vi "Direct DAC Control.vi"() -> ()   [LabVIEW 2012]
uses:
  Type/_GUI Method.ctl
  Type/_Lens Property.ctl
  Type/_Mass Range Property.ctl
  Type/_Mass Range Parameters.ctl
  Type/_RT Res Type.ctl
  Type/_Run Mode.ctl
  Type/_RT Command.ctl
  Configuration/_Global Configuration.vi
panel:
  in  "Q2DC EN":bool
  in  "Count1":dbl=400.0 caption="Lens Value" format="%#.3f"
  in  "Count2":dbl=400.0 caption="High Value" format="%#.3f"
  in  "Time1":dbl=1.0 caption="Low Dwell (ms)" format="%#.3f"
  in  "Time2":dbl=1.0 caption="High Dwell (ms)" format="%#.3f"
  in  "Scans":i32=1
  in  "Step Size":dbl=-1.0 format="%#.3f"
  in  "Unit":bool
  in  "Q1DC EN":bool
  in  "Q1 POL":bool
  in  "Q2 POL":bool
  out "DAC Value":i32=98187
  in  "Lens Table":i32(listbox)
  in  "NewMethod":bool
  in  "Method":T1={"Lenses"=[{"Scan Type"=0, "Scans"=1, "Time 1"=1.0, "Time 2"=1.0, "Value 1"=400.0, "Value 2"=400.0, "Step Size"=-1.0}, {"Scan Type"=0, "Scans"=1, "Time 1"=1.0, "Time 2"=1.0, "Value 1"=150.0, "Value 2"=150.0, "Step Size"=1.0}, {"Scan Type"=0, "Scans"=1, "Time 1"=1.0, "Time 2"=1.0, "Value 1"=32000.0, "Value 2"=32000.0, "Step Size"=1.0}, {"Scan Type"=0, "Scans"=1, "Time 1"=1.0, "Time 2"=1.0, "Value 1"=400.0, "Value 2"=400.0, "Step Size"=1.0}, {"Scan Type"=0, "Scans"=1, "Time 1"=1.0, "Time 2"=1.0, "Value 1"=150.0, "Value 2"=150.0, "Step Size"=1.0}, {"Scan Type"=0, "Scans"=1, "Time 1"=1.0, "Time 2"=1.0, "Value 1"=64000.0, "Value 2"=64000.0, "Step Size"=1.0}, {"Scan Type"=0, "Scans"=1, "Time 1"=1.0, "Time 2"=1.0, "Value 1"=420.0, "Value 2"=420.0, "Step Size"=1.0}, {"Scan Type"=0, "Scans"=1, "Time 1"=1.0, "Time 2"=1.0, "Value 1"=30.0, "Value 2"=30.0, "Step Size"=1.0}, {"Scan Type"=0, "Scans"=1, "Time 1"=1.0, "Time 2"=1.0, "Value 1"=15.0, "Value 2"=15.0, "Step Size"=1.0}, {"Scan Type"=0, "Scans"=1, "Time 1"=1.0, "Time 2"=1.0, "Value 1"=0.0, "Value 2"=0.0, "Step Size"=1.0}, {"Scan Type"=0, "Scans"=1, "Time 1"=1.0, "Time 2"=1.0, "Value 1"=0.0, "Value 2"=0.0, "Step Size"=1.0}, {"Scan Type"=0, "Scans"=1, "Time 1"=1.0, "Time 2"=1.0, "Value 1"=0.0, "Value 2"=0.0, "Step Size"=1.0}, {"Scan Type"=0, "Scans"=1, "Time 1"=1.0, "Time 2"=1.0, "Value 1"=0.0, "Value 2"=0.0, "Step Size"=1.0}, {"Scan Type"=0, "Scans"=1, "Time 1"=1.0, "Time 2"=1.0, "Value 1"=0.0, "Value 2"=0.0, "Step Size"=1.0}, {"Scan Type"=0, "Scans"=1, "Time 1"=1.0, "Time 2"=1.0, "Value 1"=-0.5, "Value 2"=-0.5, "Step Size"=1.0}, {"Scan Type"=0, "Scans"=1, "Time 1"=1.0, "Time 2"=1.0, "Value 1"=-2.0, "Value 2"=-2.0, "Step Size"=1.0}, {"Scan Type"=0, "Scans"=1, "Time 1"=1.0, "Time 2"=1.0, "Value 1"=-1.2, "Value 2"=-1.2, "Step Size"=1.0}, {"Scan Type"=0, "Scans"=1, "Time 1"=1.0, "Time 2"=1.0, "Value 1"=0.0, "Value 2"=0.0, "Step Size"=1.0}, {"Scan Type"=0, "Scans"=1, "Time 1"=1.0, "Time 2"=1.0, "Value 1"=-240.0, "Value 2"=-240.0, "Step Size"=1.0}, {"Scan Type"=0, "Scans"=1, "Time 1"=1.0, "Time 2"=1.0, "Value 1"=-50.0, "Value 2"=-50.0, "Step Size"=1.0}, {"Scan Type"=0, "Scans"=1, "Time 1"=1.0, "Time 2"=1.0, "Value 1"=-52.0, "Value 2"=-52.0, "Step Size"=1.0}, {"Scan Type"=0, "Scans"=1, "Time 1"=1.0, "Time 2"=1.0, "Value 1"=-100.0, "Value 2"=-100.0, "Step Size"=1.0}, {"Scan Type"=0, "Scans"=1, "Time 1"=1.0, "Time 2"=1.0, "Value 1"=-54.0, "Value 2"=-54.0, "Step Size"=1.0}, {"Scan Type"=0, "Scans"=1, "Time 1"=1.0, "Time 2"=1.0, "Value 1"=-400.0, "Value 2"=-400.0, "Step Size"=1.0}, {"Scan Type"=0, "Scans"=1, "Time 1"=1.0, "Time 2"=1.0, "Value 1"=30.0, "Value 2"=30.0, "Step Size"=1.0}, {"Scan Type"=0, "Scans"=1, "Time 1"=1.0, "Time 2"=1.0, "Value 1"=2000.0, "Value 2"=2000.0, "Step Size"=1.0}, {"Scan Type"=0, "Scans"=1, "Time 1"=1.0, "Time 2"=1.0, "Value 1"=-6000.0, "Value 2"=-6000.0, "Step Size"=1.0}, {"Scan Type"=0, "Scans"=1, "Time 1"=1.0, "Time 2"=1.0, "Value 1"=0.0, "Value 2"=0.0, "Step Size"=1.0}, {"Scan Type"=0, "Scans"=1, "Time 1"=1.0, "Time 2"=1.0, "Value 1"=0.0, "Value 2"=0.0, "Step Size"=1.0}, {"Scan Type"=0, "Scans"=1, "Time 1"=1.0, "Time 2"=1.0, "Value 1"=250.0, "Value 2"=250.0, "Step Size"=1.0}, {"Scan Type"=0, "Scans"=1, "Time 1"=1.0, "Time 2"=1.0, "Value 1"=-250.0, "Value 2"=-250.0, "Step Size"=1.0}, {"Scan Type"=0, "Scans"=1, "Time 1"=1.0, "Time 2"=1.0, "Value 1"=250.0, "Value 2"=250.0, "Step Size"=1.0}, {"Scan Type"=0, "Scans"=1, "Time 1"=1.0, "Time 2"=1.0, "Value 1"=-250.0, "Value 2"=-250.0, "Step Size"=1.0}, {"Scan Type"=0, "Scans"=1, "Time 1"=1.0, "Time 2"=1.0, "Value 1"=500.0, "Value 2"=500.0, "Step Size"=1.0}, {"Scan Type"=0, "Scans"=1, "Time 1"=1.0, "Time 2"=1.0, "Value 1"=-500.0, "Value 2"=-500.0, "Step Size"=1.0}, {"Scan Type"=0, "Scans"=1, "Time 1"=1.0, "Time 2"=1.0, "Value 1"=0.55, "Value 2"=0.55, "Step Size"=1.0}, {"Scan Type"=0, "Scans"=1, "Time 1"=1.0, "Time 2"=1.0, "Value 1"=0.0, "Value 2"=0.0, "Step Size"=1.0}, {"Scan Type"=0, "Scans"=1, "Time 1"=1.0, "Time 2"=1.0, "Value 1"=100.0, "Value 2"=100.0, "Step Size"=1.0}, {"Scan Type"=0, "Scans"=1, "Time 1"=1.0, "Time 2"=1.0, "Value 1"=0.0, "Value 2"=0.0, "Step Size"=1.0}, {"Scan Type"=0, "Scans"=1, "Time 1"=1.0, "Time 2"=1.0, "Value 1"=5.0, "Value 2"=5.0, "Step Size"=1.0}, {"Scan Type"=0, "Scans"=1, "Time 1"=1.0, "Time 2"=1.0, "Value 1"=0.0, "Value 2"=0.0, "Step Size"=1.0}, {"Scan Type"=0, "Scans"=1, "Time 1"=1.0, "Time 2"=1.0, "Value 1"=0.0, "Value 2"=0.0, "Step Size"=1.0}, {"Scan Type"=0, "Scans"=1, "Time 1"=1.0, "Time 2"=1.0, "Value 1"=100.0, "Value 2"=100.0, "Step Size"=1.0}, {"Scan Type"=0, "Scans"=1, "Time 1"=1.0, "Time 2"=1.0, "Value 1"=0.0, "Value 2"=0.0, "Step Size"=1.0}, {"Scan Type"=0, "Scans"=1, "Time 1"=1.0, "Time 2"=1.0, "Value 1"=5.0, "Value 2"=5.0, "Step Size"=1.0}, {"Scan Type"=0, "Scans"=1, "Time 1"=1.0, "Time 2"=1.0, "Value 1"=5000.0, "Value 2"=5000.0, "Step Size"=1.0}, {"Scan Type"=0, "Scans"=1, "Time 1"=1.0, "Time 2"=1.0, "Value 1"=0.0, "Value 2"=0.0, "Step Size"=1.0}, {"Scan Type"=0, "Scans"=1, "Time 1"=1.0, "Time 2"=1.0, "Value 1"=100.0, "Value 2"=100.0, "Step Size"=1.0}, {"Scan Type"=0, "Scans"=1, "Time 1"=1.0, "Time 2"=1.0, "Value 1"=0.0, "Value 2"=0.0, "Step Size"=1.0}, {"Scan Type"=0, "Scans"=1, "Time 1"=1.0, "Time 2"=1.0, "Value 1"=5.0, "Value 2"=5.0, "Step Size"=1.0}, {"Scan Type"=0, "Scans"=1, "Time 1"=1.0, "Time 2"=1.0, "Value 1"=1000.0, "Value 2"=1000.0, "Step Size"=1.0}, {"Scan Type"=0, "Scans"=1, "Time 1"=1.0, "Time 2"=1.0, "Value 1"=1.0, "Value 2"=1.0, "Step Size"=1.0}], "Mass Ranges"=[], "Acquire"=FALSE, "MCA"=FALSE, "Q1DC EN"=FALSE, "Q1 POL"=FALSE, "Q3 POL"=FALSE, "Q1 RF  EN"=FALSE, "Averaging"=FALSE, "Log Scale"=FALSE, "CPS"=FALSE, "Unit"=FALSE, "Data Path"=path "", "Run Mode"=enum."MRM (Q1/Q2)", "Fixed Mass (amu)"=0.0, "Q3DC EN"=FALSE, "Q3 RF  EN"=FALSE, "Negative"=FALSE} {"Mass Ranges"."Res" items=["High/High", "Medium/Medium", "Low/Low", "High/Medium", "High/Low", "Medium/High", "Medium/Low", "Low/High", "Low/Medium"]}
  in  "BloUpdate":bool
  # "Selected Lens Property"
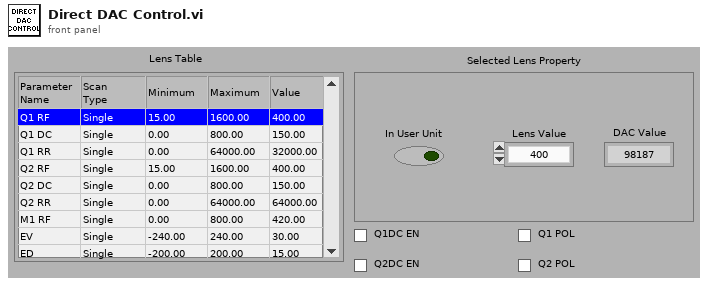
[diagram p1: front panel]
types:
  T1 = typedef "_GUI Method.ctl" = cluster{"Lenses":T2[], "Mass Ranges":T3[], "Acquire":bool, "MCA":bool, "Q1DC EN":bool, "Q1 POL":bool, "Q3 POL":bool, "Q1 RF  EN":bool, "Averaging":bool, "Log Scale":bool, "CPS":bool, "Unit":bool, "Data Path":path, "Run Mode":T6, "Fixed Mass (amu)":dbl, "Q3DC EN":bool, "Q3 RF  EN":bool, "Negative":bool}
  T2 = typedef "_Lens Property.ctl" = cluster{"Scan Type":u8, "Scans":i32, "Time 1":dbl, "Time 2":dbl, "Value 1":dbl, "Value 2":dbl, "Step Size":dbl}
  T3 = typedef "_Mass Range Property.ctl" = cluster{"Start":dbl, "Stop":dbl, "Step Size":dbl, "Steps":i32, "Dwell":dbl, "Parameters":T4[], "Res":T5}
  T4 = typedef "_Mass Range Parameters.ctl" = cluster{"Name":string, "Ch#":u8, "StartV":dbl, "StopV":dbl, "StepV":dbl, "Index":u8}
  T5 = typedef "_RT Res Type.ctl" = u16
  T6 = typedef "_Run Mode.ctl" = enum16{"MRM (Q1/Q2)", "Q1 Scan", "Q1 SRM", "Q2 Scan", "Q2 SRM", "Product Scan", "Precursor Scan", "Neutral Loss", "Neutral Gain"}
  T7 = typedef "_RT Command.ctl" = enum16{"Start", "Stop", "Runtime Update", "Get Data", "Get Info", "Get Status", "Get Param", "Get Config", "Get Table", "Read ADC", "Set Oscillator", "Update Config", "Update Table", "Set All Pol", "Set Pol and DC", "Set Max Mass", "Toggle RP", "Toggle EL", "Set PIC", "Initialize Turbo", "Send Turbo Comm", "Close Turbo", "P1", "P2", "P3", "Send Serial", "Set LC Out", "Get LC In", "Read VAC", "Test Table", "Toggle Power", "Get Startup", "Set Startup", "Get ADC Table", "Set ADC Table", "Get Brief Status", "Get Detail Status", "Auxiliary Update", "Set CC Logics", "Set CC Input Logics", "Ignore Error"}
  T8 = typedef "_RT Instrument 2.ctl" = cluster{"Table":T9[], "Instrument":string[]}
  T9 = typedef "_RT Configuration 2.ctl" = cluster{"Name":string, "Ch#":u8, "Min":dbl, "Max":dbl, "Def+":dbl, "Def-":dbl, "Offset":dbl, "Slope":dbl, "Type":u8, "Description":string, "SettleT":dbl}
  T10 = cluster{"Scan Type":u8, "Unit":bool, "Count1":dbl, "Count2":dbl, "Time1":dbl, "Time2":dbl, "Scans":i32, "Step Size":dbl, "Lens Table":i32}
  T11 = cluster{"Scan Type":u8, "Unit":bool, "Count1":dbl, "Count2":dbl, "Time1":dbl, "Time2":dbl, "Scans":i32, "Step Size":dbl, "Start DAC":i32, "Ramp Time (ms)":i32}
  T12 = cluster{bool, "Value 1":dbl, "Value 2":dbl, "Step Size":dbl}
  T13 = cluster{"Unit":bool, "Count1":dbl, "Count2":dbl, "Step Size":dbl}
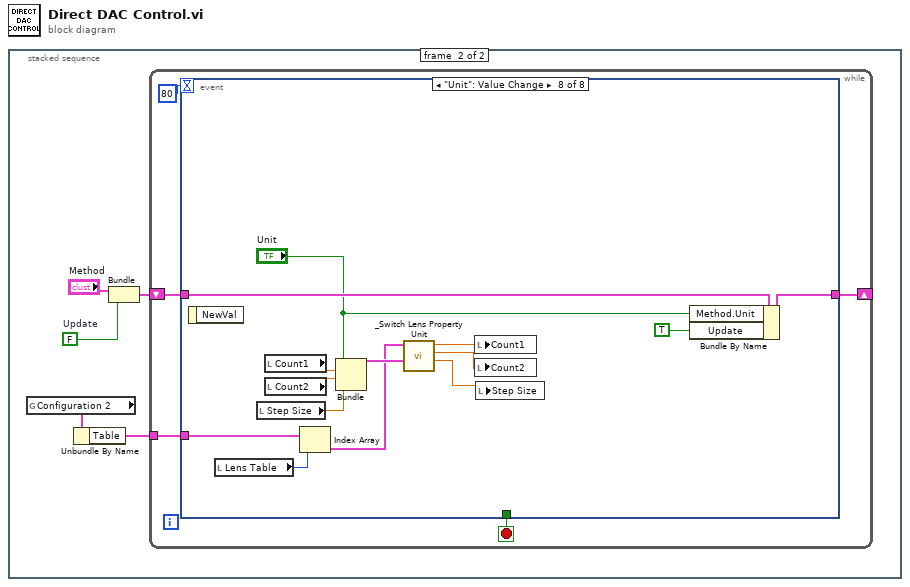
[diagram p0: block diagram]
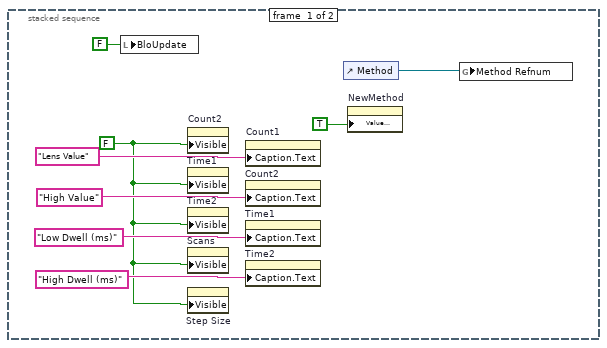
[diagram p2: hidden frame]
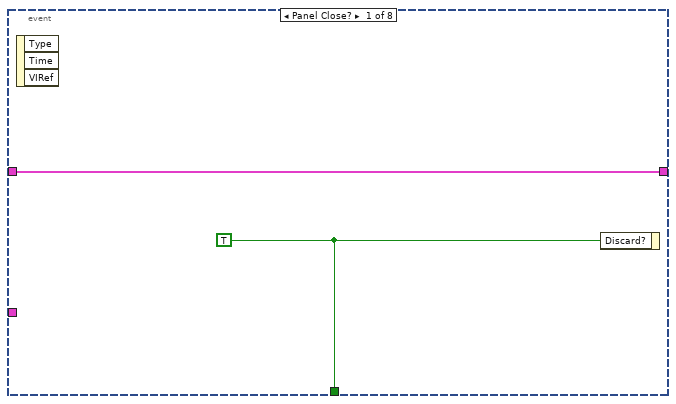
[diagram p3: hidden frame]
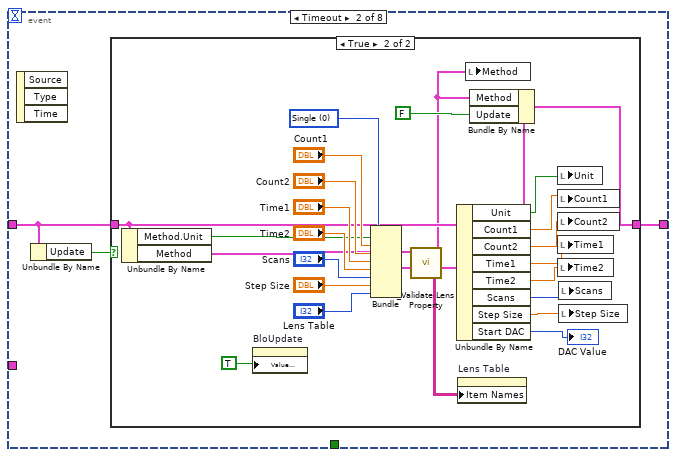
[diagram p4: hidden frame]
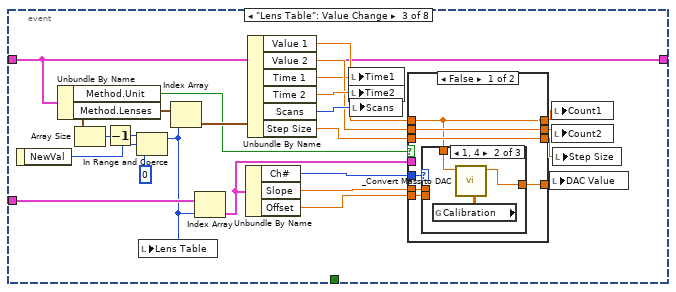
[diagram p6: hidden frame]
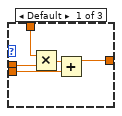
[diagram p7: hidden frame]
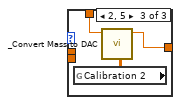
[diagram p8: hidden frame]
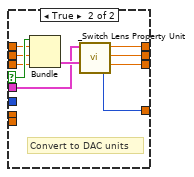
[diagram p9: hidden frame]
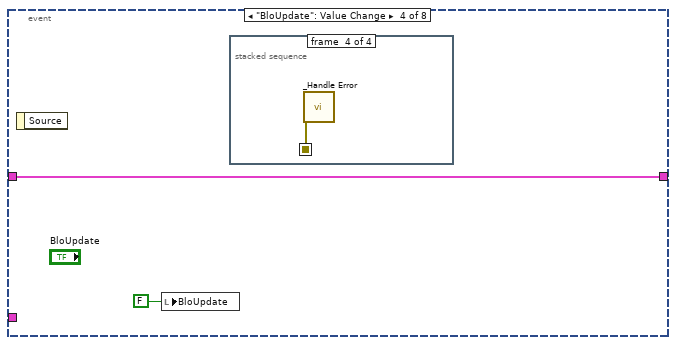
[diagram p10: hidden frame]
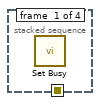
[diagram p11: hidden frame]
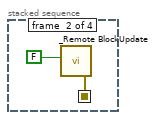
[diagram p12: hidden frame]
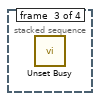
[diagram p13: hidden frame]
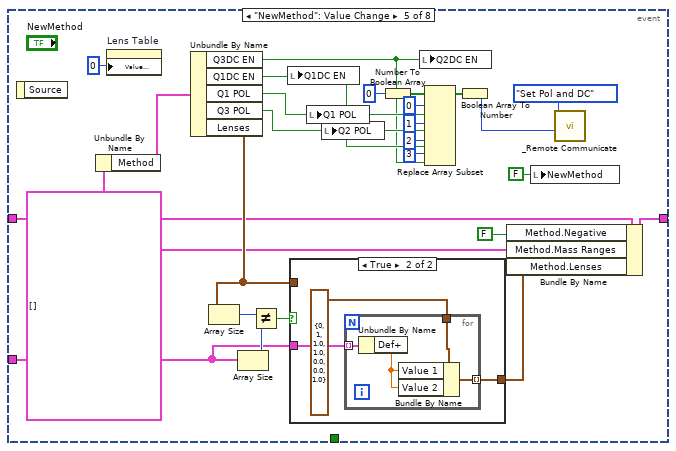
[diagram p14: hidden frame]
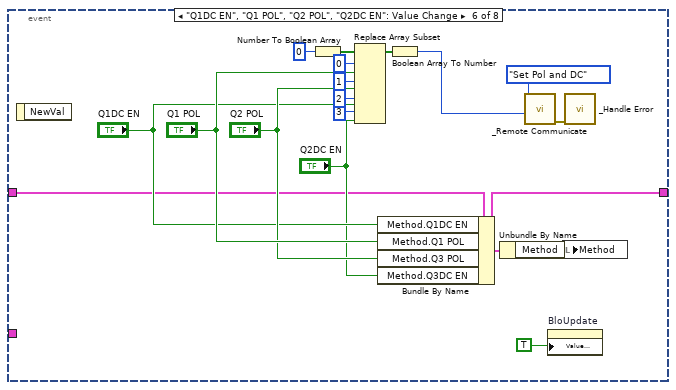
[diagram p16: hidden frame]
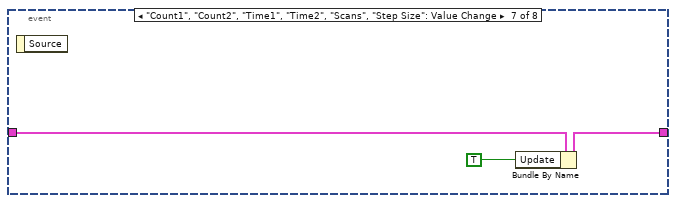
[diagram p17: hidden frame]
diagram:
  n1 = stacked-sequence {
    frame #0 {
      w1 = FALSE
      n2 = local write "BloUpdate"(FALSE ("Unit")) -> ()
      n3 = property on="Count2" class="DigNum (strict)"("Visible"=w1) -> ()  [unwired: 2 in, 2 out]
      n4 = property on="Time1" class="DigNum (strict)"("Visible"=w1) -> ()  [unwired: 2 in, 2 out]
      n5 = property on="Time2" class="DigNum (strict)"("Visible"=w1) -> ()  [unwired: 2 in, 2 out]
      n6 = property on="Scans" class="DigNum (strict)"("Visible"=w1) -> ()  [unwired: 2 in, 2 out]
      n7 = property on="Step Size" class="DigNum (strict)"("Visible"=w1) -> ()  [unwired: 2 in, 2 out]
      n8 = property on="Count1" class="DigNum (strict)"("Caption.Text"="Lens Value") -> ()  [unwired: 2 in, 2 out]
      n9 = property on="Count2" class="DigNum (strict)"("Caption.Text"="High Value") -> ()  [unwired: 2 in, 2 out]
      n10 = property on="Time1" class="DigNum (strict)"("Caption.Text"="Low Dwell (ms)") -> ()  [unwired: 2 in, 2 out]
      n11 = property on="Time2" class="DigNum (strict)"("Caption.Text"="High Dwell (ms)") -> ()  [unwired: 2 in, 2 out]
      n12 = control-ref of="Method"() -> (w6:refnum<vi>)
      n13 = property on="NewMethod" class="Bool (strict)"("Value (Signaling)"=TRUE ("Visible")) -> ()  [unwired: 2 in, 2 out]
      n14 = global write "_Global Configuration.vi" "Method Refnum"(w6) -> ()
    }
    frame #1 {
      w12 = FALSE  # Update
      n15 = global read "_Global Configuration.vi" "Configuration 2"() -> (w10:T8)
      n16 = Unbundle By Name(w10) -> ("Table"=w9:T9[])
      n17 = Bundle("Method"="Method", "Update"=w12) -> (w11:cluster{"Method":T1, "Update":bool})  [unwired: 1 out]
      n18 = while {
        shift-right: [w15] -> _
        shift-left: w11 -> [w17]
        tunnel: w9 -> [w14]
        stop <- w18 stop-if-true
        n19 = event shown="[7] \"Unit\": Value Change" {
          selector: _ -> [_ _ _ _ _ _ _ _]
          dyn-events: _ -> [_ _ _ _ _ _ _ _]
          timeout: 80 -> [_ _ _ _ _ _ _ _]
          tunnel: [w20 _ _ _ _ _ _ _] -> w18
          tunnel: w17 -> [w19 w22 w61 w103 w122 w145 w161 w165]
          tunnel: [w19 w23 w61 w103 w121 w158 w160 w164] -> w15
          tunnel: w14 -> [_ _ w59 _ w125 _ _ w169]
          event Panel Close? {
            w20 = TRUE ("Discard?")
            n20 = event-data() -> ()  [unwired: 4 out]
            n21 = event-data("Discard?"=w20) -> ()  [unwired: 1 in, 1 out]
          }
          event Timeout {
            n22 = event-data() -> ()  [unwired: 4 out]
            n23 = Unbundle By Name(w22) -> ("Update"=w21:bool)
            n24 = case shown="True" w21 {
              tunnel: w22 -> [w24 w35]
              tunnel: [w24 w33] -> w23
              frame False {
              }
              frame True {
                w50 = u8 0 items=["Single", "Dual", "Ramp"] ("Scan Type")
                n25 = Unbundle By Name(w35) -> ("Method.Unit"=w32:bool, "Method"=w36:T1)
                n26 = property on="BloUpdate" class="Bool (strict)"("Value (Signaling)"=TRUE) -> ()  [unwired: 2 in, 2 out]
                n27 = Bundle("Scan Type"=w50, "Unit"=w32, "Count1"="Count1", "Count2"="Count2", "Time1"="Time1", "Time2"="Time2", "Scans"="Scans", "Step Size"="Step Size", "Lens Table"="Lens Table") -> (w43:T10)  [unwired: 1 out]
                n28 = call "_Validate Lens Property.vi"("Lens Property In"=w43, "Method In"=w36) -> ("Lens Table"=w37:string[][], "Lens Property Out"=w42:T11, "Method Out"=w30:T1)  [unwired: 2 in, 2 out]
                n29 = Unbundle By Name(w42) -> ("Unit"=w31:bool, "Count1"=w40:dbl, "Count2"=w39:dbl, "Time1"=w25:dbl, "Time2"=w26:dbl, "Scans"=w38:i32, "Step Size"=w41:dbl, "Start DAC"=→"DAC Value":i32)
                n30 = property on="Lens Table" class="MCListbox (strict)"("Item Names"=w37) -> ()  [unwired: 2 in, 2 out]
                n31 = local write "Method"(w30) -> ()
                n32 = Bundle By Name(cluster=w35, "Method"=w30, "Update"=FALSE) -> (w33:cluster{"Method":T1, "Update":bool})
                n33 = local write "Unit"(w31) -> ()
                n34 = local write "Count1"(w40) -> ()
                n35 = local write "Count2"(w39) -> ()
                n36 = local write "Time1"(w25) -> ()
                n37 = local write "Time2"(w26) -> ()
                n38 = local write "Scans"(w38) -> ()
                n39 = local write "Step Size"(w41) -> ()
              }
            }
          }
          event "Lens Table": Value Change {
            n40 = event-data() -> ("NewVal"=w66:i32)  [unwired: 1 out]
            n41 = Unbundle By Name(w61) -> ("Method.Unit"=w51:bool, "Method.Lenses"=w62:T2[])
            n42 = Array Size(array=w62) -> (size(s)=w63:i32)
            n43 = Decrement(x=w63) -> (x-1=w64:i32)
            n44 = In Range and Coerce(upper limit=w64, x=w66, lower limit=0) -> (coerced(x)=w58:i32)  [unwired: 1 out]
            n45 = local write "Lens Table"(w58) -> ()
            n46 = Index Array(array=w62, index=w58) -> (element=w60:T2)
            n47 = Index Array(array=w59, index=w58) -> (element=w54:T9)
            n48 = Unbundle By Name(w54) -> ("Ch#"=w57:u8, "Slope"=w56:dbl, "Offset"=w55:dbl)
            n49 = Unbundle By Name(w60) -> ("Value 1"=w70:dbl, "Value 2"=w69:dbl, "Time 1"=w68:dbl, "Time 2"=w74:dbl, "Scans"=w73:i32, "Step Size"=w71:dbl)
            n50 = local write "Time1"(w68) -> ()
            n51 = local write "Time2"(w74) -> ()
            n52 = local write "Scans"(w73) -> ()
            n53 = case shown="False" w51 {
              selector: w51 -> [_ w99]
              tunnel: w71 -> [w80 w95]
              tunnel: w69 -> [w81 w96]
              tunnel: w70 -> [w78 w98]
              tunnel: [w78 w102] -> w52
              tunnel: [w81 w101] -> w72
              tunnel: [w80 w100] -> w53
              tunnel: [w77 w94] -> w67
              tunnel: w57 -> [w79 _]
              tunnel: w56 -> [w76 _]
              tunnel: w55 -> [w75 _]
              tunnel: w54 -> [_ w93]
              frame False {
                n54 = case shown="1, 4" w79 {
                  tunnel: w78 -> [w85 w88 w91]
                  tunnel: [w82 w87 w90] -> w77
                  tunnel: w76 -> [w84 _ _]
                  tunnel: w75 -> [w83 _ _]
                  frame Default {
                    n55 = Multiply(x=w85, y=w84) -> (x*y=w86:dbl)
                    n56 = Add(x=w86, y=w83) -> (x+y=w82:dbl)
                  }
                  frame 1, 4 {
                    n57 = global read "_Global Configuration.vi" "Calibration"() -> (w89:dbl[][])
                    n58 = call "_Convert Mass to DAC.vi"("Calibration Table"=w89, "Mass"=w88) -> ("DAC Value"=w87:dbl)  [unwired: 2 in, 3 out]
                  }
                  frame 2, 5 {
                    n59 = global read "_Global Configuration.vi" "Calibration 2"() -> (w92:dbl[][])
                    n60 = call "_Convert Mass to DAC.vi"("Calibration Table"=w92, "Mass"=w91) -> ("DAC Value"=w90:dbl)  [unwired: 2 in, 3 out]
                  }
                }
              }
              frame True {
                # "Convert to DAC units"
                n61 = Bundle(w99, "Value 1"=w98, "Value 2"=w96, "Step Size"=w95) -> (w97:T12)  [unwired: 1 out]
                n62 = call "_Switch Lens Property Unit.vi"("Lens Property In"=w97, "Configuration"=w93) -> ("DAC Value"=w94:i32, "Step Size"=w100:dbl, "Count2"=w101:dbl, "Count1"=w102:dbl)  [unwired: 1 in, 1 out]
              }
            }
            n63 = local write "DAC Value"(w67) -> ()
            n64 = local write "Count1"(w52) -> ()
            n65 = local write "Count2"(w72) -> ()
            n66 = local write "Step Size"(w53) -> ()
          }
          event "BloUpdate": Value Change {
            n67 = event-data() -> ()  [unwired: 2 out]
            n68 = local write "BloUpdate"(FALSE) -> ()
            n69 = stacked-sequence {
              seq-local: [_ w106 _ _] -> [_ _ _ w107]
              frame #0 {
                n70 = call <vilib>:"Set Busy.vi"() -> ()  [unwired: 4 in, 8 out]
              }
              frame #1 {
                n71 = call "_Remote BlockUpdate.vi"("Filter (T)"=FALSE) -> ("error out"=w106:errorcluster)  [unwired: 2 in, 4 out]
              }
              frame #2 {
                n72 = call <vilib>:"Unset Busy.vi"() -> ()  [unwired: 2 in, 10 out]
              }
              frame #3 {
                n73 = call "_Handle Error.vi"("error in (no error)"=w107) -> ()  [unwired: 2 in, 5 out]
              }
            }
          }
          event "NewMethod": Value Change {
            n74 = event-data() -> ()  [unwired: 2 out]
            n75 = Unbundle By Name(w122) -> ("Method"=w124:T1)
            n76 = property on="Lens Table" class="MCListbox (strict)"("Value (Signaling)"=0) -> ()  [unwired: 2 in, 2 out]
            n77 = Unbundle By Name(w124) -> ("Q3DC EN"=w119:bool, "Q1DC EN"=w132:bool, "Q1 POL"=w131:bool, "Q3 POL"=w130:bool, "Lenses"=w126:T2[])
            n78 = Array Size(array=w126) -> (size(s)=w128:i32)
            n79 = Array Size(array=w125) -> (size(s)=w129:i32)
            n80 = Not Equal?(x=w128, y=w129) -> (x != y?=w127:bool)
            n81 = local write "Q1DC EN"(w132) -> ()
            n82 = case shown="True" w127 {
              tunnel: w125 -> [_ w137]
              tunnel: [w134 w135] -> w123
              tunnel: w126 -> [w134 _]
              frame False {
              }
              frame True {
                n83 = for {
                  tunnel: w137 -> [w140] mode=indexing
                  tunnel: T2 {"Scan Type"=0, "Scans"=1, "Time 1"=1.0, "Time 2"=1.0, "Value 1"=0.0, "Value 2"=0.0, "Step Size"=1.0} ("Lenses") -> [w141]
                  tunnel: [w138] -> w135 mode=indexing
                  n84 = Unbundle By Name(w140) -> ("Def+"=w139:dbl)
                  n85 = Bundle By Name(cluster=w141, "Value 1"=w139, "Value 2"=w139) -> (w138:T2)
                }
              }
            }
            n86 = local write "Q1 POL"(w131) -> ()
            n87 = local write "Q2 POL"(w130) -> ()
            n88 = Number To Boolean Array(number=u16 0) -> (Boolean array=w115:bool[])
            n89 = local write "Q2DC EN"(w119) -> ()
            n90 = Replace Array Subset(array=w115, new element #1=w131, index #1=0 ("index"), new element #2=w130, index #2=1 ("index"), new element #3=w132, index #3=2 ("index"), new element #4=w119, index #4=3 ("index")) -> (w110:bool[])
            n91 = Boolean Array To Number(Boolean array=w110) -> (number=w109:u16)
            n92 = Bundle By Name(cluster=w122, "Method.Negative"=FALSE, "Method.Mass Ranges"=T3[] [], "Method.Lenses"=w123) -> (w121:cluster{"Method":T1, "Update":bool})
            n93 = local write "NewMethod"(FALSE) -> ()
            n94 = call "_Remote Communicate.vi"("DC Param"=w109, "Command"=_RT_Command."Set Pol and DC") -> ()  [unwired: 4 in, 4 out]
          }
          event "Q1DC EN", "Q1 POL", "Q2 POL", "Q2DC EN": Value Change {
            n95 = event-data() -> ()  [unwired: 2 out]
            n96 = Number To Boolean Array(number=u16 0) -> (Boolean array=w156:bool[])
            n97 = Replace Array Subset(array=w156, new element #1="Q1 POL", index #1=0 ("index"), new element #2="Q2 POL", index #2=1 ("index"), new element #3="Q1DC EN", index #3=2 ("index"), new element #4="Q2DC EN", index #4=3 ("index")) -> (w147:bool[])
            n98 = Bundle By Name(cluster=w145, "Method.Q1DC EN"="Q1DC EN", "Method.Q1 POL"="Q1 POL", "Method.Q3 POL"="Q2 POL", "Method.Q3DC EN"="Q2DC EN") -> (w158:cluster{"Method":T1, "Update":bool})
            n99 = Boolean Array To Number(Boolean array=w147) -> (number=w146:u16)
            n100 = Unbundle By Name(w158) -> ("Method"=w159:T1)
            n101 = call "_Remote Communicate.vi"("DC Param"=w146, "Command"=_RT_Command."Set Pol and DC") -> ("error out"=w143:errorcluster)  [unwired: 4 in, 3 out]
            n102 = property on="BloUpdate" class="Bool (strict)"("Value (Signaling)"=TRUE) -> ()  [unwired: 2 in, 2 out]
            n103 = local write "Method"(w159) -> ()
            n104 = call "_Handle Error.vi"("error in (no error)"=w143) -> ()  [unwired: 2 in, 5 out]
          }
          event "Count1", "Count2", "Time1", "Time2", "Scans", "Step Size": Value Change {
            n105 = event-data() -> ()  [unwired: 2 out]
            n106 = Bundle By Name(cluster=w161, "Update"=TRUE) -> (w160:cluster{"Method":T1, "Update":bool})
          }
          event "Unit": Value Change {
            n107 = event-data() -> ()  [unwired: 2 out]
            n108 = local read "Lens Table"() -> (w168:i32)
            n109 = local read "Step Size"() -> (w176:dbl)
            n110 = local read "Count1"() -> (w175:dbl)
            n111 = local read "Count2"() -> (w174:dbl)
            n112 = Index Array(array=w169, index=w168) -> (element=w167:T9)
            n113 = Bundle("Unit"="Unit", "Count1"=w175, "Count2"=w174, "Step Size"=w176) -> (w173:T13)  [unwired: 1 out]
            n114 = call "_Switch Lens Property Unit.vi"("Lens Property In"=w173, "Configuration"=w167) -> ("Step Size"=w170:dbl, "Count2"=w171:dbl, "Count1"=w172:dbl)  [unwired: 1 in, 2 out]
            n115 = local write "Count1"(w172) -> ()
            n116 = local write "Count2"(w171) -> ()
            n117 = local write "Step Size"(w170) -> ()
            n118 = Bundle By Name(cluster=w165, "Method.Unit"="Unit", "Update"=TRUE) -> (w164:cluster{"Method":T1, "Update":bool})
          }
        }
      }
    }
  }
